vi "GLB_WebService_Status.vi"() -> ()   [LabVIEW 2018]
panel:
  out "WebService_Status":bool
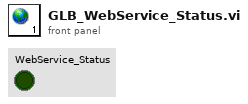
[diagram p1: front panel]
diagram:
